vi "Snake tick.vi"(8 "error in (no error)":errorcluster, 11 "Snake in":refnum<class "Snake.lvclass">) -> (0 "error out":errorcluster, 3 "Snake out":refnum<class "Snake.lvclass">)   [LabVIEW 2019, in "Snake.lvclass"]
uses:
  Snake.lvclass
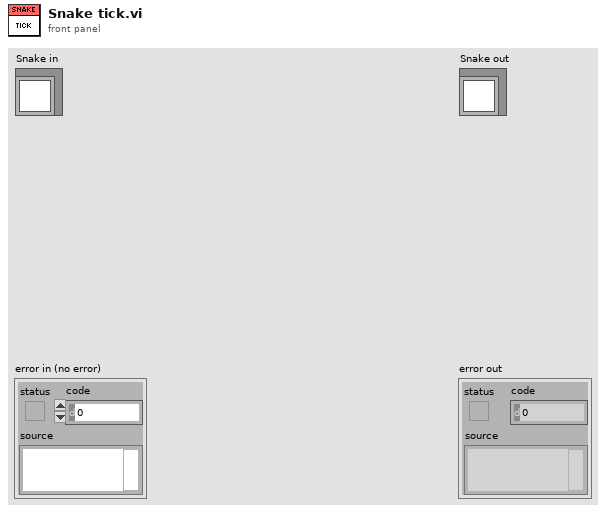
[diagram p1: front panel]
types:
  T1 = typedef "Direction STYP.ctl" = enum16{"Up", "Down", "Left", "Right"}
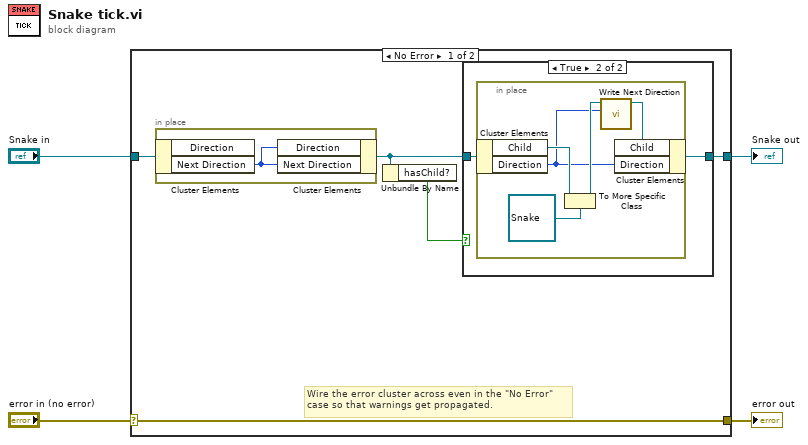
[diagram p0: block diagram]
diagram:
  n1 = case shown="No Error" "error in (no error)" {
    selector: "error in (no error)" -> [w9 w20]
    tunnel: [w9 w20] -> w3
    tunnel: [w7 w19] -> w1
    tunnel: "Snake in" -> [w8 w19]
    frame No Error {
      # "Wire the error cluster across even in the \"No Error\"\ncase so that warnings get propagated."
      n2 = in-place {
        n3 = in-place-cluster #1(w8) -> ("Next Direction"=w18:T1)  [unwired: 1 out]
        n4 = in-place-cluster #1("Direction"=w18, "Next Direction"=w18) -> (w6:refnum<class "Snake.lvclass">)
      }
      n5 = Unbundle By Name(w6) -> ("hasChild?"=w5:bool)
      n6 = case shown="True" w5 {
        tunnel: [w10 w11] -> w7
        tunnel: w6 -> [w10 w12]
        frame False {
        }
        frame True {
          n7 = in-place {
            n8 = in-place-cluster #2(w12) -> ("Child"=w17:refnum<class>, "Direction"=w13:T1)
            n9 = To More Specific Class(target class=refnum<class "Snake.lvclass"> refnum ("Snake.lvclass"), reference=w17) -> (specific class reference=w15:refnum<class "Snake.lvclass">)  [unwired: 1 in, 1 out]
            n10 = call-dynamic "Write Next Direction.vi"("Direction"=w13, "Snake in"=w15) -> ("Snake out"=w14:refnum<class "Snake.lvclass">)  [unwired: 8 in, 1 out]
            n11 = in-place-cluster #2("Child"=w14, "Direction"=w13) -> (w11:refnum<class "Snake.lvclass">)
          }
        }
      }
    }
    frame Error {
    }
  }
  "error out" <- w3
  "Snake out" <- w1
